vi "save channels to separate tiff series.vi"(8 "frame number in":i32, 9 "last frame":bool, 11 "image data in":dbl[][](array[numeric])) -> ()   [LabVIEW 2012]
doc: "SciScan 1.2 160622"
uses:
  Custom Controls/file format type def.ctl
  GFG/GFGpathGet.vi
  GFG/GFGnumericGet.vi
  GFG/GFGstringGet.vi
  GFG/GFG library.lvlib
  Libtiff3/libtiff3.llb/libtiff3.lvlib
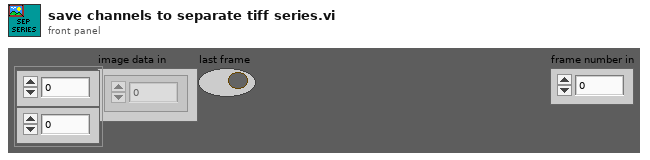
[diagram p1: front panel]
types:
  T1 = typedef "file format type def.ctl" = enum16{"16bit raw", "32bit raw", "16bit multi-tiff (interleave)", "16bit multi-tiff (separate)", "16bit multi-tiff (stacked)", "32bit multi-tiff (interleave)", "32bit multi-tiff (separate)", "32bit multi-tiff (stacked)", "16bit tiff series (interleave)", "16bit tiff series (separate)", "16bit tiff series (stacked)", "32bit tiff series (interleave)", "32bit tiff series (separate)", "32bit tiff series (stacked)"}
  T2 = cluster{"no..of.frames.to.acquire":dbl, "x.pixels":dbl, "y.pixels":dbl, "x.pixel.sz":dbl, "y.pixel.sz":dbl}
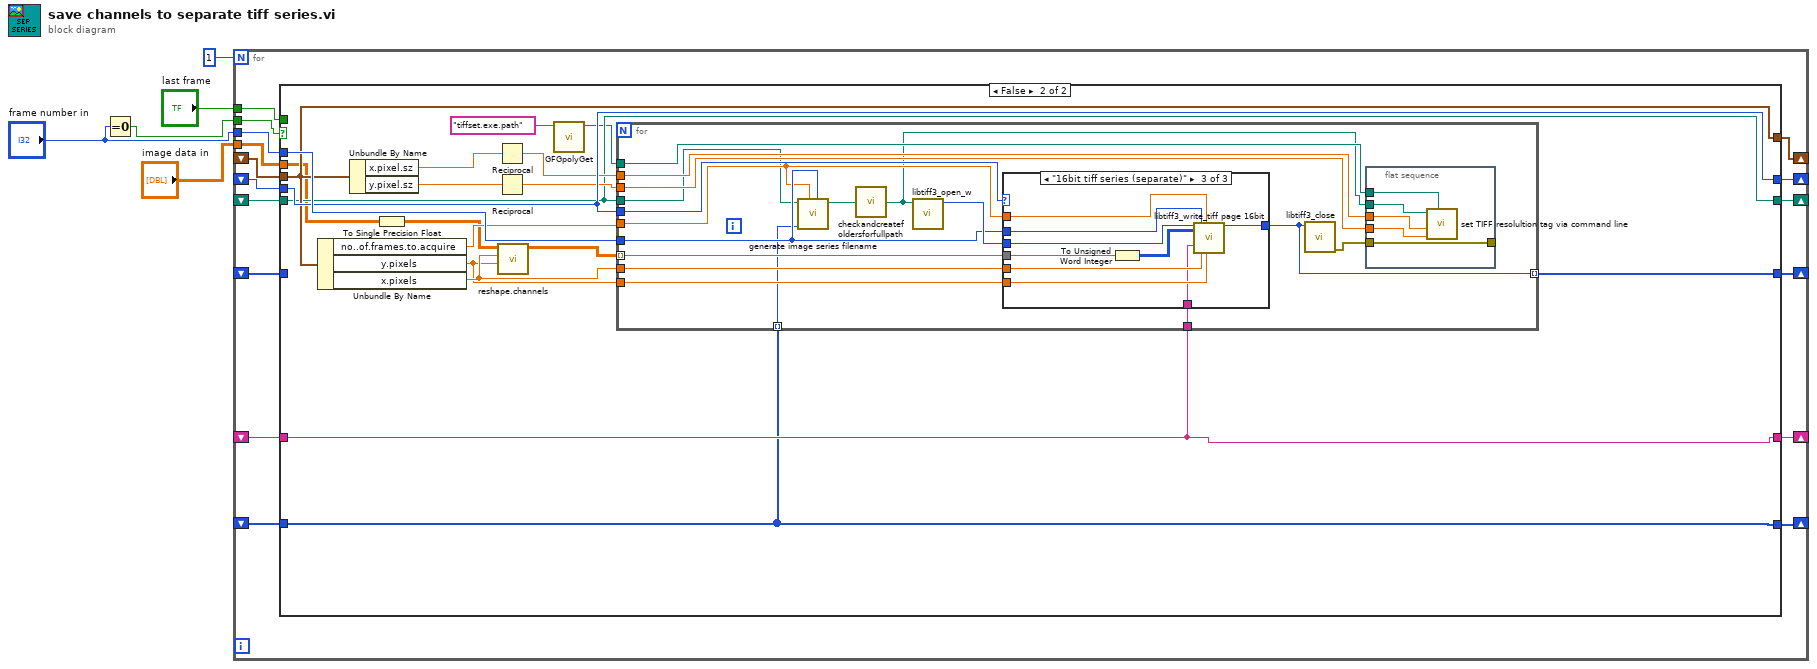
[diagram p0: block diagram]
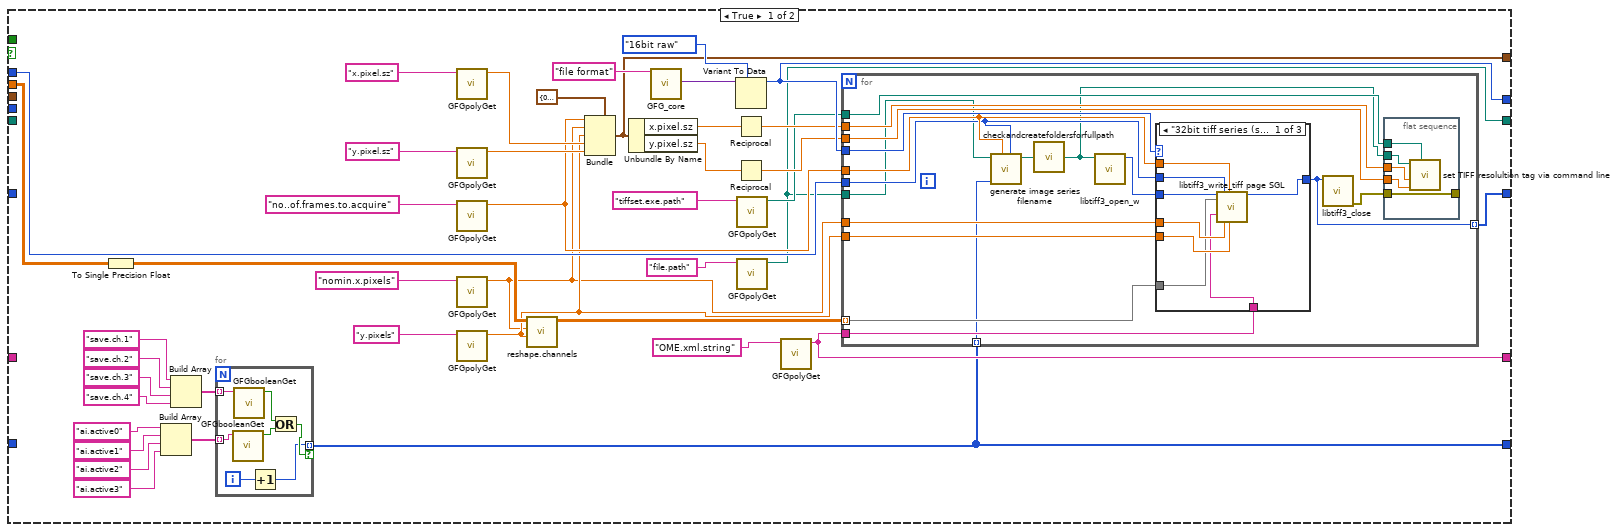
[diagram p2: hidden frame]
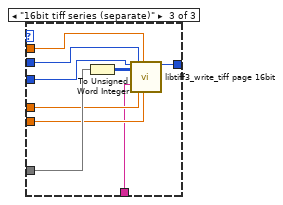
[diagram p4: hidden frame]
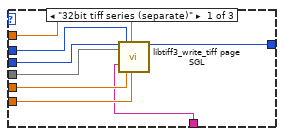
[diagram p5: hidden frame]
diagram:
  n1 = Equal To 0?(x="frame number in") -> (x = 0?=w4:bool)
  n2 = for {
    N: 1 -> [_]
    tunnel: w4 -> [w21]
    shift-right: [w20] -> _
    shift-left: _ -> [w19]
    tunnel: "image data in" -> [w18]
    shift-right: [w17] -> _
    shift-left: _ -> [w16]
    shift-right: [w15] -> _
    shift-left: _ -> [w14]
    shift-right: [w13] -> _
    shift-left: _ -> [w12]
    tunnel: "last frame" -> [w11]
    tunnel: "frame number in" -> [w10]
    shift-right: [w9] -> _
    shift-left: _ -> [w8]
    shift-right: [w7] -> _
    shift-left: _ -> [w6]
    n3 = case shown="False" w21 {
      tunnel: w16 -> [_ w127]
      tunnel: [w48 w125] -> w20
      tunnel: w19 -> [_ _]
      tunnel: w18 -> [w38 w116]
      tunnel: [w51 w127] -> w17
      tunnel: [w47 w126] -> w15
      tunnel: w14 -> [_ w126]
      tunnel: [w40 w119] -> w13
      tunnel: w12 -> [_ w119]
      tunnel: w11 -> [_ _]
      tunnel: w10 -> [w49 w129]
      tunnel: [w33 w112] -> w9
      tunnel: w8 -> [_ w112]
      tunnel: [w22 w111] -> w7
      tunnel: w6 -> [_ w111]
      frame True {
        n4 = To Single Precision Float(number=w38) -> (single precision float=w39:sgl[][])
        n5 = Build Array("ai.active0" ("Variable Name in"), "ai.active1" ("Variable Name in"), "ai.active2" ("Variable Name in"), "ai.active3" ("Variable Name in")) -> (w23:string[])
        n6 = Build Array("save.ch.1" ("Variable Name in"), "save.ch.2" ("Variable Name in"), "save.ch.3" ("Variable Name in"), "save.ch.4" ("Variable Name in")) -> (w28:string[])
        n7 = for {
          tunnel: w28 -> [w70] mode=indexing
          tunnel: w23 -> [w69] mode=indexing
          tunnel: [w64] -> w22 mode=indexing if=w65
          i -> [w66]
          n8 = call "GFGbooleanGet.vi"("Variable Name in"=w69) -> ("Boolean Value OUT"=w68:bool)  [unwired: 9 in, 1 out]
          n9 = call "GFGbooleanGet.vi"("Variable Name in"=w70) -> ("Boolean Value OUT"=w67:bool)  [unwired: 9 in, 1 out]
          n10 = Increment(x=w66) -> (x+1=w64:i32)
          n11 = Or(x=w67, y=w68) -> (x .or. y?=w65:bool)
        }
        n12 = call-poly "GFGpolyGet.vi"("Variable Name in"="x.pixel.sz" ("Tag in")) -> ("Numeric"=w54:dbl)  [unwired: 8 in, 2 out]
        n13 = call-poly "GFGpolyGet.vi"("Variable Name in"="y.pixel.sz" ("Tag in")) -> ("Numeric"=w53:dbl)  [unwired: 8 in, 2 out]
        n14 = call-poly "GFGpolyGet.vi"("Variable Name in"="no..of.frames.to.acquire") -> ("Numeric"=w50:dbl)  [unwired: 8 in, 2 out]
        n15 = call-poly "GFGpolyGet.vi"("Variable Name in"="nomin.x.pixels" ("Tag in")) -> ("Numeric"=w35:dbl)  [unwired: 8 in, 2 out]
        n16 = call-poly "GFGpolyGet.vi"("Variable Name in"="y.pixels" ("Tag in")) -> ("Numeric"=w36:dbl)  [unwired: 8 in, 2 out]
        n17 = call "reshape.channels.vi"("y.pixels"=w36, "x.pixels"=w35, "element"=w39) -> ("Array"=w37:dbl[][][])  [unwired: 8 in]
        n18 = Bundle(cluster=T2 {"no..of.frames.to.acquire"=0.0, "x.pixels"=0.0, "y.pixels"=0.0, "x.pixel.sz"=0.0, "y.pixel.sz"=0.0} ("output cluster"), "no..of.frames.to.acquire"=w50, "x.pixels"=w35, "y.pixels"=w36, "x.pixel.sz"=w54, "y.pixel.sz"=w53) -> (w47:T2)
        n19 = Unbundle By Name(w47) -> ("x.pixel.sz"=w43:dbl, "y.pixel.sz"=w44:dbl)
        n20 = call "GFG_core.vi"("Variable Name in"="file format") -> ("Variant Out"=w62:variant)  [unwired: 12 in, 6 out]
        n21 = Variant To Data(type=file_format_type_def."16bit raw" ("file format"), Variant=w62) -> (data=w51:T1)  [unwired: 1 in, 1 out]
        n22 = Reciprocal(x=w43) -> (1/x=w45:dbl)
        n23 = Reciprocal(x=w44) -> (1/x=w46:dbl)
        n24 = call-poly "GFGpolyGet.vi"("Variable Name in"="tiffset.exe.path") -> ("Path"=w41:path)  [unwired: 8 in, 2 out]
        n25 = call-poly "GFGpolyGet.vi"("Variable Name in"="file.path") -> ("Path"=w40:path)  [unwired: 8 in, 2 out]
        n26 = call-poly "GFGpolyGet.vi"("Variable Name in"="OME.xml.string") -> ("String"=w33:string)  [unwired: 9 in, 1 out]
        n27 = for {
          tunnel: w51 -> [w87]
          tunnel: w35 -> [w85]
          tunnel: w36 -> [w84]
          tunnel: w50 -> [w82]
          tunnel: w49 -> [w81]
          tunnel: [w80] -> w48 mode=indexing
          tunnel: w46 -> [w78]
          tunnel: w45 -> [w77]
          tunnel: w41 -> [w76]
          tunnel: w40 -> [w75]
          tunnel: w37 -> [w74] mode=indexing
          tunnel: w33 -> [w72]
          tunnel: w22 -> [w71] mode=indexing
          n28 = call "generate image series filename.vi"("frame number in"=w81, "no..of.frames.to.acquire"=w82, "channel"=w71, "Path IN"=w75) -> ("appended path"=w83:path)  [unwired: 7 in]
          n29 = call "checkandcreatefoldersforfullpath.vi"("Path IN"=w83) -> ("Path OUT"=w73:path)  [unwired: 4 in]
          n30 = call "libtiff3_open_w.vi"("Input path"=w73) -> ("handle"=w86:i32)  [unwired: 9 in, 1 out]
          n31 = case shown="\"32bit tiff series (separate)\"" w87 {
            tunnel: w74 -> [w94 _ w107]
            tunnel: w86 -> [w97 w101 w108]
            tunnel: w81 -> [w98 _ w109]
            tunnel: w82 -> [w99 _ w110]
            tunnel: [w100 w101 w103] -> w80
            tunnel: w85 -> [w95 _ w105]
            tunnel: w84 -> [w96 _ w104]
            tunnel: w72 -> [w93 _ w102]
            frame "32bit tiff series (separate)" {
              n32 = call "libtiff3_write_tiff page SGL.vi"("Handle"=w97, "Image Pixels (Float)"=w94, "Image Description"=w93, "page"=w98, "x.pixels"=w95, "totalpages"=w99, "y.pixels"=w96) -> ("Handle out"=w100:i32)  [unwired: 11 in, 1 out]
            }
            frame Default {
            }
            frame "16bit tiff series (separate)" {
              n33 = To Unsigned Word Integer(number=w107) -> (unsigned 16bit integer=w106:u16[][])
              n34 = call "libtiff3_write_tiff page 16bit.vi"("Handle"=w108, "Image Pixels (U16)"=w106, "ImageDescription"=w102, "page"=w109, "x.pixels"=w105, "totalpages"=w110, "y.pixels"=w104) -> ("Handle out"=w103:i32)  [unwired: 11 in, 1 out]
            }
          }
          n35 = call "libtiff3_close.vi"("Handle"=w80) -> ("error out"=w79:errorcluster)  [unwired: 9 in]
          n36 = flat-sequence {
            tunnel: w79 -> [w90]
            tunnel: w77 -> [w92]
            tunnel: w78 -> [w91]
            tunnel: [w90] -> _
            tunnel: w76 -> [w89]
            tunnel: w73 -> [w88]
            frame #0 {
              n37 = call "set TIFF resolultion tag via command line.vi"("tiffset.exe file path"=w89, "y pixels per m"=w91, "x pixels per m"=w92, "TIFF file path"=w88) -> ()  [unwired: 8 in]
            }
          }
        }
      }
      frame False {
        n38 = Unbundle By Name(w126) -> ("no..of.frames.to.acquire"=w128:dbl, "y.pixels"=w117:dbl, "x.pixels"=w118:dbl)
        n39 = Unbundle By Name(w126) -> ("x.pixel.sz"=w121:dbl, "y.pixel.sz"=w122:dbl)
        n40 = To Single Precision Float(number=w116) -> (single precision float=w115:sgl[][])
        n41 = Reciprocal(x=w121) -> (1/x=w123:dbl)
        n42 = Reciprocal(x=w122) -> (1/x=w124:dbl)
        n43 = call "reshape.channels.vi"("y.pixels"=w117, "x.pixels"=w118, "element"=w115) -> ("Array"=w114:dbl[][][])  [unwired: 8 in]
        n44 = call-poly "GFGpolyGet.vi"("Variable Name in"="tiffset.exe.path") -> ("Path"=w113:path)  [unwired: 8 in, 2 out]
        n45 = for {
          tunnel: w129 -> [w144]
          tunnel: w128 -> [w143]
          tunnel: w127 -> [w142]
          tunnel: w117 -> [w141]
          tunnel: w118 -> [w140]
          tunnel: [w139] -> w125 mode=indexing
          tunnel: w124 -> [w137]
          tunnel: w123 -> [w136]
          tunnel: w119 -> [w135]
          tunnel: w114 -> [w134] mode=indexing
          tunnel: w113 -> [w133]
          tunnel: w112 -> [w131]
          tunnel: w111 -> [w130] mode=indexing
          n46 = call "generate image series filename.vi"("frame number in"=w144, "no..of.frames.to.acquire"=w143, "channel"=w130, "Path IN"=w135) -> ("appended path"=w145:path)  [unwired: 7 in]
          n47 = call "checkandcreatefoldersforfullpath.vi"("Path IN"=w145) -> ("Path OUT"=w132:path)  [unwired: 4 in]
          n48 = call "libtiff3_open_w.vi"("Input path"=w132) -> ("handle"=w146:i32)  [unwired: 9 in, 1 out]
          n49 = case shown="\"16bit tiff series (separate)\"" w142 {
            tunnel: w134 -> [w153 _ w166]
            tunnel: w146 -> [w156 w160 w167]
            tunnel: w144 -> [w157 _ w168]
            tunnel: w143 -> [w158 _ w169]
            tunnel: [w159 w160 w162] -> w139
            tunnel: w140 -> [w154 _ w164]
            tunnel: w141 -> [w155 _ w163]
            tunnel: w131 -> [w152 _ w161]
            frame "32bit tiff series (separate)" {
              n50 = call "libtiff3_write_tiff page SGL.vi"("Handle"=w156, "Image Pixels (Float)"=w153, "Image Description"=w152, "page"=w157, "x.pixels"=w154, "totalpages"=w158, "y.pixels"=w155) -> ("Handle out"=w159:i32)  [unwired: 11 in, 1 out]
            }
            frame Default {
            }
            frame "16bit tiff series (separate)" {
              n51 = To Unsigned Word Integer(number=w166) -> (unsigned 16bit integer=w165:u16[][])
              n52 = call "libtiff3_write_tiff page 16bit.vi"("Handle"=w167, "Image Pixels (U16)"=w165, "ImageDescription"=w161, "page"=w168, "x.pixels"=w164, "totalpages"=w169, "y.pixels"=w163) -> ("Handle out"=w162:i32)  [unwired: 11 in, 1 out]
            }
          }
          n53 = call "libtiff3_close.vi"("Handle"=w139) -> ("error out"=w138:errorcluster)  [unwired: 9 in]
          n54 = flat-sequence {
            tunnel: w138 -> [w149]
            tunnel: w136 -> [w151]
            tunnel: w137 -> [w150]
            tunnel: [w149] -> _
            tunnel: w133 -> [w148]
            tunnel: w132 -> [w147]
            frame #0 {
              n55 = call "set TIFF resolultion tag via command line.vi"("tiffset.exe file path"=w148, "y pixels per m"=w150, "x pixels per m"=w151, "TIFF file path"=w147) -> ()  [unwired: 8 in]
            }
          }
        }
      }
    }
  }
